vi "Get Metric.vi"(8 "error in (no error)":errorcluster, 10 "Metric Name":string, 11 "Session Handle in":T1) -> (0 "error out":errorcluster, 1 "Found Metric?":bool, 2 "Metric":refnum<data-value>, 3 "Session Handle out":T1)   [LabVIEW 2020, in "Registry.lvlib" / "Registry Session.lvclass"]
uses:
  Registry Session.lvclass
  Typedefs/Session Handle.ctl
  metrics/metric/Metric.lvclass
  Registry Session.lvclass/Registry Session.ctl
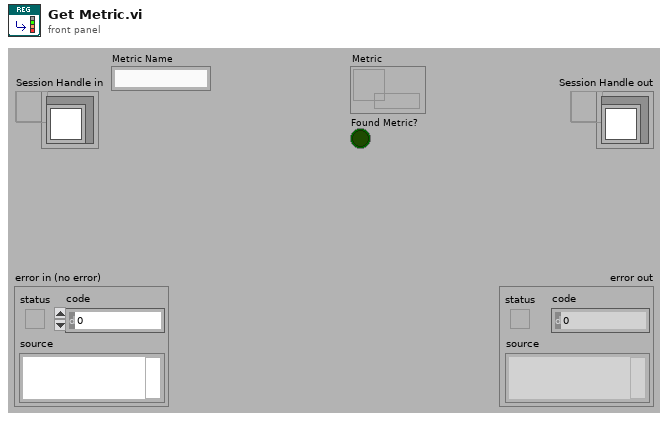
[diagram p1: front panel]
types:
  T1 = typedef "Registry.lvlib/Registry Session.lvclass/Session Handle.ctl" = refnum<data-value>
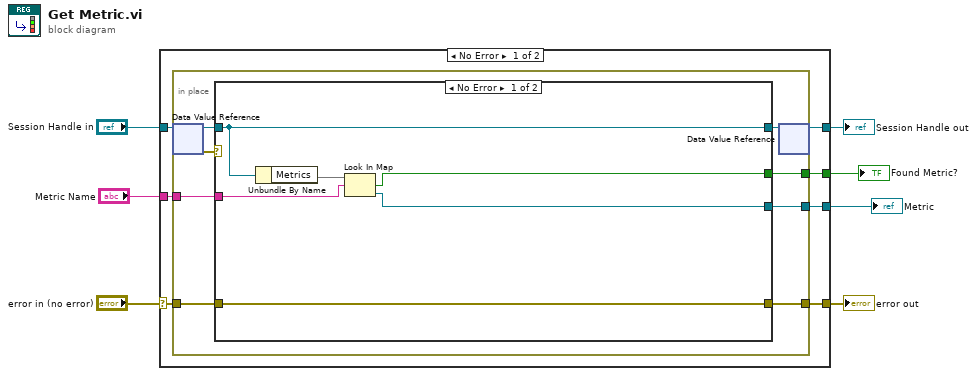
[diagram p0: block diagram]
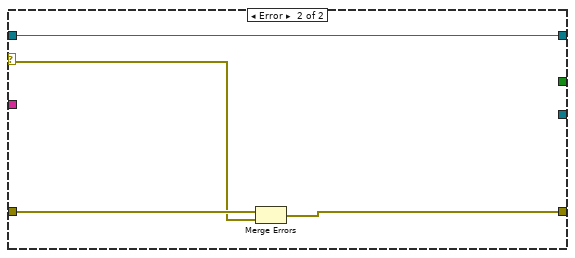
[diagram p2: hidden frame]
diagram:
  n1 = case shown="No Error" "error in (no error)" {
    selector: "error in (no error)" -> [w12 w33]
    tunnel: "Session Handle in" -> [w14 w34]
    tunnel: [w13 w34] -> w6
    tunnel: [w11 w33] -> w5
    tunnel: "Metric Name" -> [w10 _]
    tunnel: [w9 _] -> w2
    tunnel: [w8 _] -> w1
    frame No Error {
      n2 = in-place {
        in-place-border: w12 -> [w18]
        in-place-border: [w21] -> w11
        in-place-border: w10 -> [w17]
        in-place-border: [w16] -> w9
        in-place-border: [w15] -> w8
        n3 = in-place-dvr #1(w14) -> (w22:refnum<class "Registry Session.lvclass">, w19:errorcluster)
        n4 = case shown="No Error" w19 {
          selector: w19 -> [_ w31]
          tunnel: w22 -> [w23 w29]
          tunnel: [w24 w30] -> w21
          tunnel: [w23 w29] -> w20
          tunnel: w18 -> [w24 w32]
          tunnel: w17 -> [w27 _]
          tunnel: [w26 _] -> w16
          tunnel: [w25 _] -> w15
          frame No Error {
            n5 = Unbundle By Name(w23) -> ("Metrics"=w28:map{string, refnum<data-value>})
            n6 = Look In Map(map=w28, key=w27) -> (key not found?=w25:bool, value=w26:refnum<data-value>)  [unwired: 1 in]
          }
          frame Error {
            n7 = Merge Errors(w32, w31) -> (w30:errorcluster)
          }
        }
        n8 = in-place-dvr #1(w20) -> (w13:T1)  [unwired: 1 out]
      }
    }
    frame Error {
    }
  }
  "Session Handle out" <- w6
  "error out" <- w5
  "Metric" <- w2
  "Found Metric?" <- w1
